vi "LoadMethodInfo.vi"(1 "ViRef":refnum<vi>, 5 "error in (no error)":errorcluster) -> (15 "ExecutionInfo":T2, 16 "Descriptions":T1, 19 "error out":errorcluster)   [LabVIEW 2018, in "Executer.lvclass"]
uses:
  Executer.lvclass
  typedefs/MethodExecutionInfo.ctl
  typedefs/MethodDescription.ctl
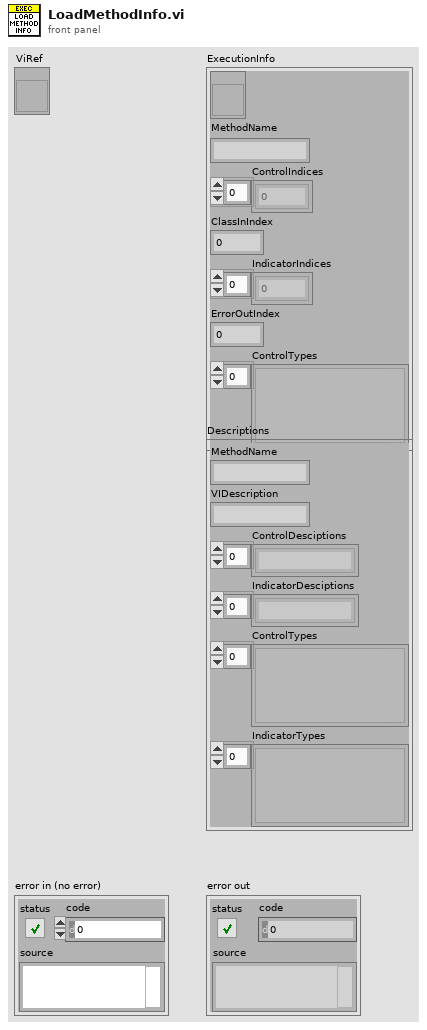
[diagram p1: front panel]
types:
  T1 = typedef "Executer.lvclass/MethodDescription.ctl" = cluster{"MethodName":string, "VIDescription":string, "ControlDesciptions":string[], "IndicatorDesciptions":string[], "ControlTypes":variant[], "IndicatorTypes":variant[]}
  T2 = typedef "Executer.lvclass/MethodExecutionInfo.ctl" = cluster{"viRef":refnum<vi>, "MethodName":string, "ControlIndices":i32[], "ClassInIndex":i32, "IndicatorIndices":i32[], "ErrorOutIndex":i32, "ControlTypes":variant[]}
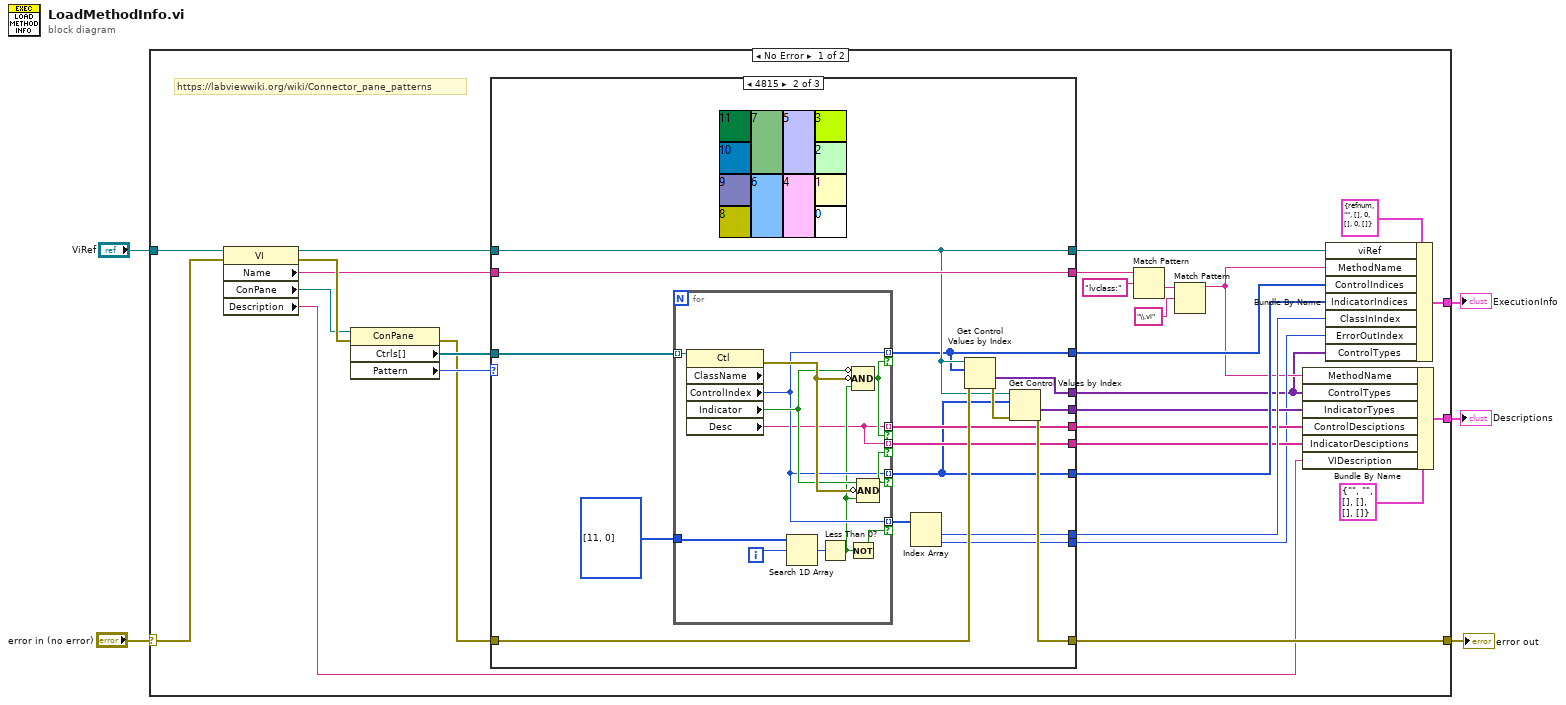
[diagram p0: block diagram]
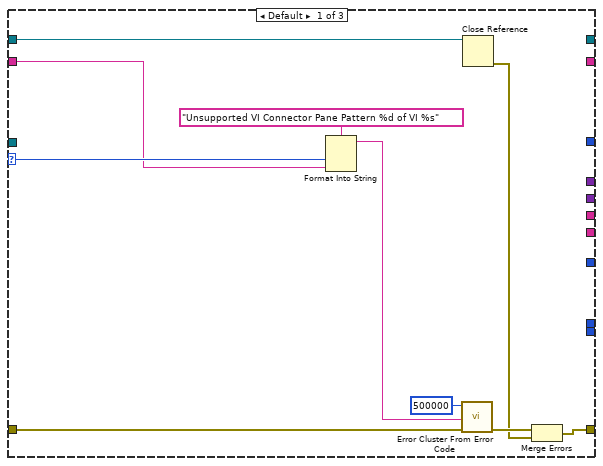
[diagram p2: hidden frame]
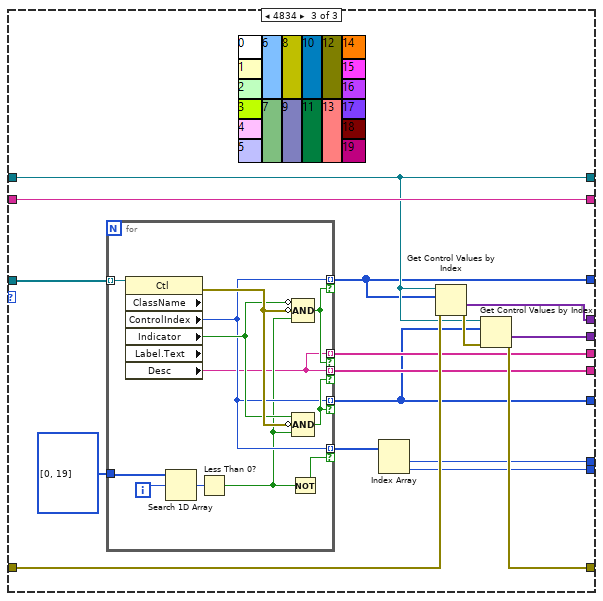
[diagram p3: hidden frame]
diagram:
  n1 = case shown="No Error" "error in (no error)" {
    selector: "error in (no error)" -> [w15 w101]
    tunnel: [w33 w101] -> w5
    tunnel: [w32 _] -> w3
    tunnel: [w31 _] -> w2
    tunnel: "ViRef" -> [w6 _]
    frame No Error {
      # "https://labviewwiki.org/wiki/Connector_pane_patterns"
      n2 = property class="VI"(reference=w6, error in=w15) -> (reference out=w27:refnum<vi>, error out=w34:errorcluster, "Name"=w22:string, "ConPane"=w29:refnum<vi>, "Description"=w14:string)
      n3 = property class="ConPane"(reference=w29, error in=w34) -> (error out=w26:errorcluster, "Ctrls[]"=w30:refnum<vi>[], "Pattern"=w28:u32)  [unwired: 1 out]
      n4 = case shown="4815" w28 {
        selector: w28 -> [w41 _ _]
        tunnel: w30 -> [_ w55 w84]
        tunnel: [_ w50 w76] -> w24
        tunnel: [_ w49 w75] -> w19
        tunnel: [_ w45 w81] -> w12
        tunnel: [w36 w59 w87] -> w33
        tunnel: w27 -> [w37 w51 w77]
        tunnel: [_ w46 w82] -> w23
        tunnel: [_ w54 w80] -> w17
        tunnel: [_ w53 w79] -> w16
        tunnel: w26 -> [w38 w58 w86]
        tunnel: w22 -> [w39 w52 w78]
        tunnel: [_ w51 w77] -> w8
        tunnel: [_ w52 w78] -> w20
        tunnel: [_ w48 w74] -> w7
        tunnel: [_ w47 w73] -> w13
        frame Default {
          n5 = Format Into String(format string="Unsupported VI Connector Pane Pattern %d of VI %s" ("error message (\"\")"), w41, w39) -> (resulting string=w40:string)  [unwired: 2 in, 1 out]
          n6 = call <vilib>:"Error Cluster From Error Code.vi"("error in (no error)"=w38, "error message (\"\")"=w40, "error code (0)"=500000) -> ("error out"=w44:errorcluster)  [unwired: 6 in]
          n7 = Close Reference(reference=w37) -> (error out=w35:errorcluster)  [unwired: 1 in]
          n8 = Merge Errors(w44, w35) -> (w36:errorcluster)
        }
        frame 4815 {
          n9 = for {
            tunnel: w55 -> [w72] mode=indexing
            tunnel: [w64] -> w49 mode=indexing if=w68
            tunnel: [w64] -> w50 mode=indexing if=w69
            tunnel: i32[] [11, 0] -> [w71]
            tunnel: [w61] -> w54 mode=indexing if=w69
            tunnel: [w61] -> w53 mode=indexing if=w68
            tunnel: [w64] -> w56 mode=indexing if=w62
            i -> [w65]
            n10 = property class="Ctl" props=["ClassName", "ControlIndex", "Indicator", "Desc"](reference=w72) -> (error out=w67:errorcluster, "ControlIndex"=w64:i32, "Indicator"=w66:bool, "Desc"=w61:string)  [unwired: 1 in, 2 out]
            n11 = Search 1D Array(1D array=w71, element=w65) -> (index of element=w70:i32)  [unwired: 1 in]
            n12 = Less Than 0?(x=w70) -> (x < 0?=w63:bool)
            n13 = Not(x=w63) -> (.not. x?=w62:bool)
            n14 = Compound Arithmetic op=AND(invert w66, invert w67, w63) -> (w69:bool)
            n15 = Compound Arithmetic op=AND(w66, invert w67, w63) -> (w68:bool)
          }
          n16 = Index Array(array=w56) -> (element #1=w46:i32, element #2=w45:i32)  [unwired: 2 in]
          n17 = Get Control Values by Index(0:w51, 1:w50, 3:w58) -> (10:w48:variant[], 11:w60:errorcluster)
          n18 = Get Control Values by Index(0:w51, 1:w49, 3:w60) -> (10:w47:variant[], 11:w59:errorcluster)
        }
        frame 4834 {
          n19 = for {
            tunnel: w84 -> [w100] mode=indexing
            tunnel: [w92] -> w75 mode=indexing if=w96
            tunnel: [w92] -> w76 mode=indexing if=w97
            tunnel: i32[] [0, 19] -> [w99]
            tunnel: [w89] -> w80 mode=indexing if=w97
            tunnel: [w89] -> w79 mode=indexing if=w96
            tunnel: [w92] -> w85 mode=indexing if=w90
            i -> [w93]
            n20 = property class="Ctl" props=["ClassName", "ControlIndex", "Indicator", "Label", "Text", "Desc"](reference=w100) -> (error out=w95:errorcluster, "ControlIndex"=w92:i32, "Indicator"=w94:bool, "Desc"=w89:string)  [unwired: 1 in, 3 out]
            n21 = Search 1D Array(1D array=w99, element=w93) -> (index of element=w98:i32)  [unwired: 1 in]
            n22 = Less Than 0?(x=w98) -> (x < 0?=w91:bool)
            n23 = Not(x=w91) -> (.not. x?=w90:bool)
            n24 = Compound Arithmetic op=AND(invert w94, invert w95, w91) -> (w97:bool)
            n25 = Compound Arithmetic op=AND(w94, invert w95, w91) -> (w96:bool)
          }
          n26 = Index Array(array=w85) -> (element #1=w82:i32, element #2=w81:i32)  [unwired: 2 in]
          n27 = Get Control Values by Index(0:w77, 1:w76, 3:w86) -> (10:w74:variant[], 11:w88:errorcluster)
          n28 = Get Control Values by Index(0:w77, 1:w75, 3:w88) -> (10:w73:variant[], 11:w87:errorcluster)
        }
      }
      n29 = Match Pattern(string=w20, regular expression="lvclass:" ("search string")) -> (after substring=w11:string)  [unwired: 1 in, 3 out]
      n30 = Match Pattern(string=w11, regular expression="\\.vi") -> (before substring=w9:string)  [unwired: 1 in, 3 out]
      n31 = Bundle By Name(cluster=T1 {"MethodName"="", "VIDescription"="", "ControlDesciptions"=[], "IndicatorDesciptions"=[], "ControlTypes"=[], "IndicatorTypes"=[]} ("Descriptions"), "MethodName"=w9, "ControlTypes"=w7, "IndicatorTypes"=w13, "ControlDesciptions"=w17, "IndicatorDesciptions"=w16, "VIDescription"=w14) -> (w31:T1)
      n32 = Bundle By Name(cluster=T2 {"viRef"=refnum, "MethodName"="", "ControlIndices"=[], "ClassInIndex"=0, "IndicatorIndices"=[], "ErrorOutIndex"=0, "ControlTypes"=[]} ("Cluster"), "viRef"=w8, "MethodName"=w9, "ControlIndices"=w24, "IndicatorIndices"=w19, "ClassInIndex"=w23, "ErrorOutIndex"=w12, "ControlTypes"=w7) -> (w32:T2)
    }
    frame Error {
    }
  }
  "error out" <- w5
  "ExecutionInfo" <- w3
  "Descriptions" <- w2
